vi "Handle MES commands.vi"(6 "Sequence Context In":refnum<k7>, 8 "error in (no error)":errorcluster, 9 "RequestData in":T2, 10 "Request":u32, 11 "Data Value Reference in":T1) -> (0 "error out":errorcluster, 1 "PLC MES Error":bool, 2 "RequestData out":T2, 3 "Data Value Reference out":T1)   [LabVIEW 2023]
uses:
  RequestData.ctl
  MessageInfo.ctl
  <vilib>/Noffz/UTP IO/UTP IO Library/methods/poly/plc/Write PLC Variable (Boolean).vi
  <vilib>/Noffz/UTP IO/UTP IO Library/methods/poly/plc/Read PLC Variable (String).vi
  <vilib>/addons/TestStand/_TSUtility.llb/TestStand - Get Property Value (String).vi
  <vilib>/addons/TestStand/_TSUtility.llb/TestStand - Set Property Value (String).vi
  <vilib>/addons/TestStand/_TSUtility.llb/TestStand - Set Property Value (Boolean).vi
  <vilib>/addons/TestStand/_TSUtility.llb/TestStand - Set Property Value (String Array).vi
  <vilib>/Noffz/UTP IO/UTP IO Library/UTP IO Pool Session.lvclass
  <vilib>/Noffz/UTP IO/UTP IO Library/methods/poly/plc/Write PLC Variable (String).vi
  <vilib>/Noffz/UTP IO/UTP IO Library/Typedefs/Session Handle.ctl
panel:
  out "Packaging Instructions":string[](array[string])
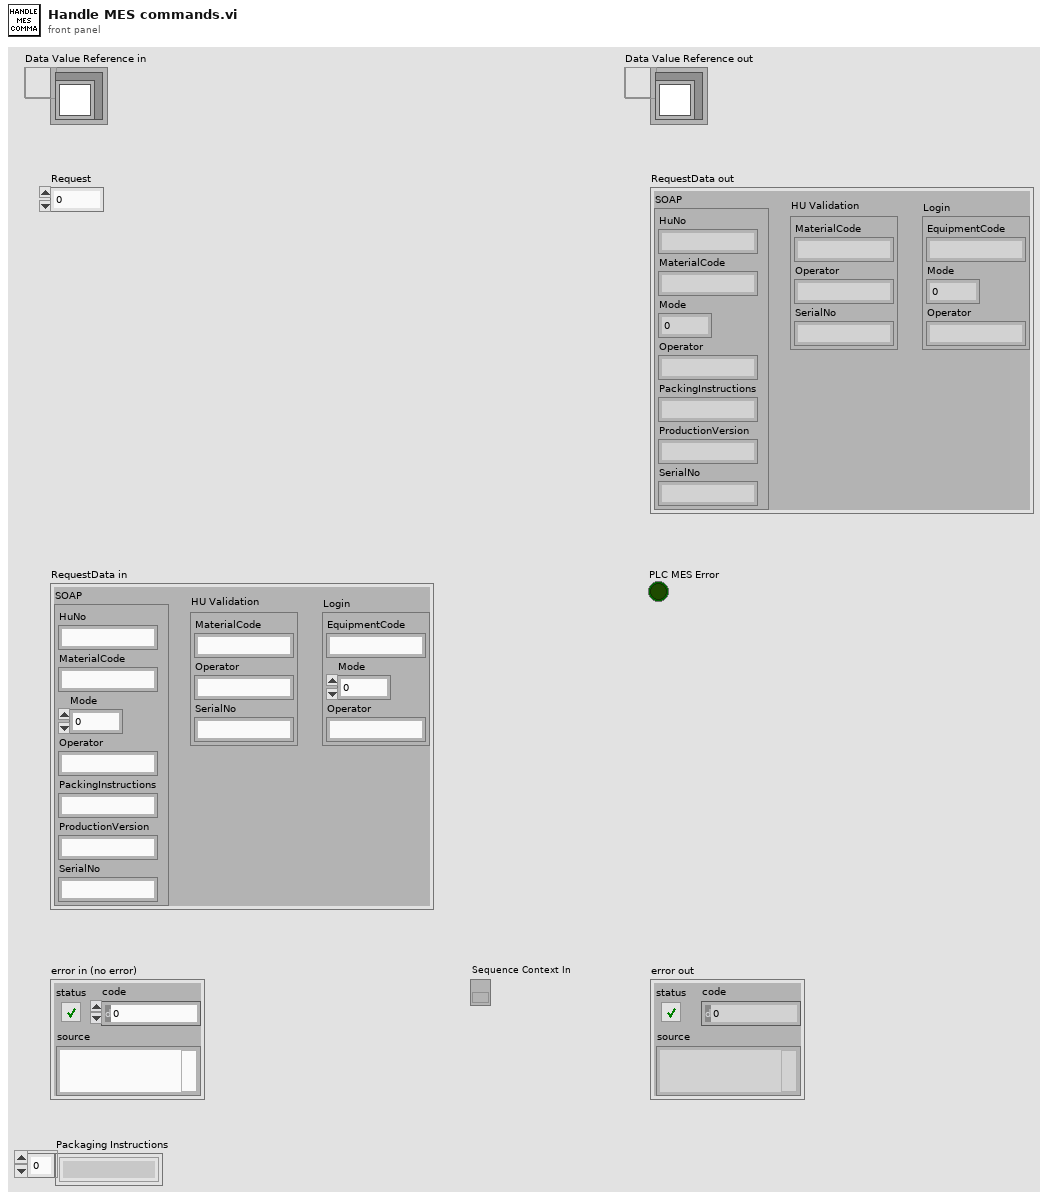
[diagram p1: front panel]
types:
  T1 = typedef "UTP IO Library.lvlib/UTP IO Pool Session.lvclass/Session Handle.ctl" = refnum<data-value>
  T2 = typedef "RequestData.ctl" = cluster{"SOAP":cluster{"HuNo":string, "MaterialCode":string, "Mode":i32, "Operator":string, "PackingInstructions":string, "ProductionVersion":string, "SerialNo":string}, "HU Validation":cluster{"MaterialCode":string, "Operator":string, "SerialNo":string}, "Login":cluster{"EquipmentCode":string, "Mode":i32, "Operator":string}}
  T3 = typedef "MessageInfo.ctl" = cluster{"Message Code":string, "Message Description":string}
  T4 = cluster{"EquipmentCode":string, "Mode":i32, "Operator":string}
  T5 = cluster{"MessageCode":string, "MessageDescription":string, "Result":string}
  T6 = cluster{"HuNo":string, "MaterialCode":string, "Mode":i32, "Operator":string, "PackingInstructions":string, "ProductionVersion":string, "SerialNo":string}
  T7 = cluster{"BoxCount":i32, "BoxNo":string, "MaxBoxCount":i32, "MaxSerialCount":i32, "MessageCode":string, "MessageDescription":string, "PackingInstruction1":string, "PackingInstruction2":string, "PackingInstruction3":string, "PackingInstruction4":string, "PackingInstruction5":string, "PalletNo":string, "Result":string, "SerialCount":i32}
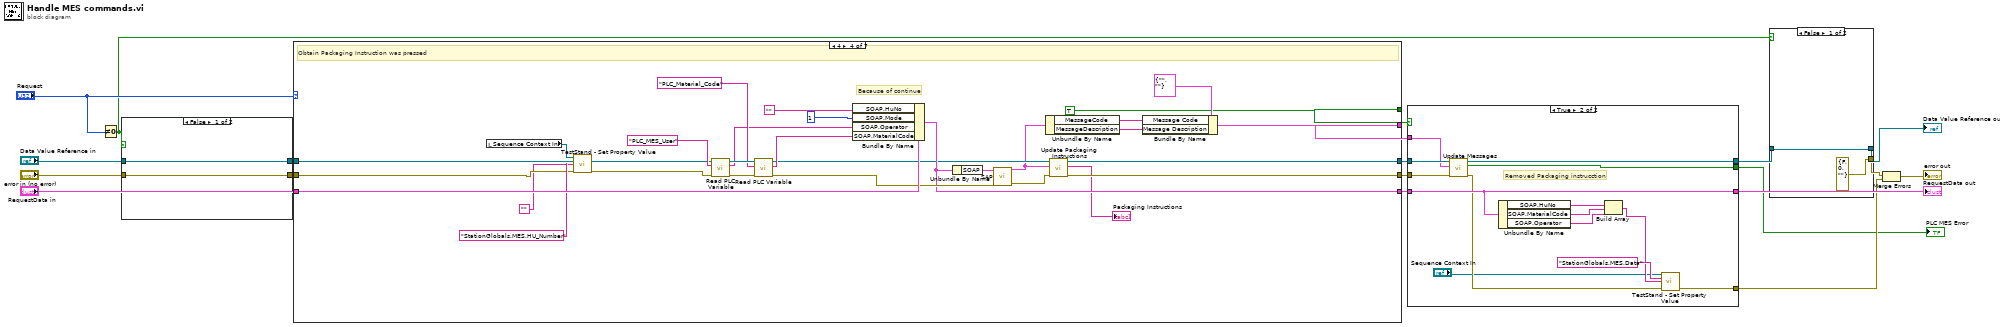
[diagram p0: block diagram]
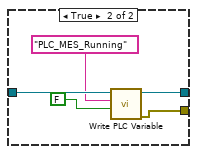
[diagram p2: hidden frame]
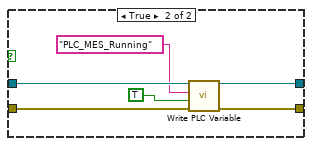
[diagram p3: hidden frame]
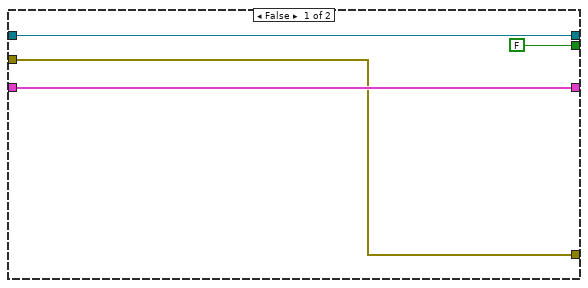
[diagram p4: hidden frame]
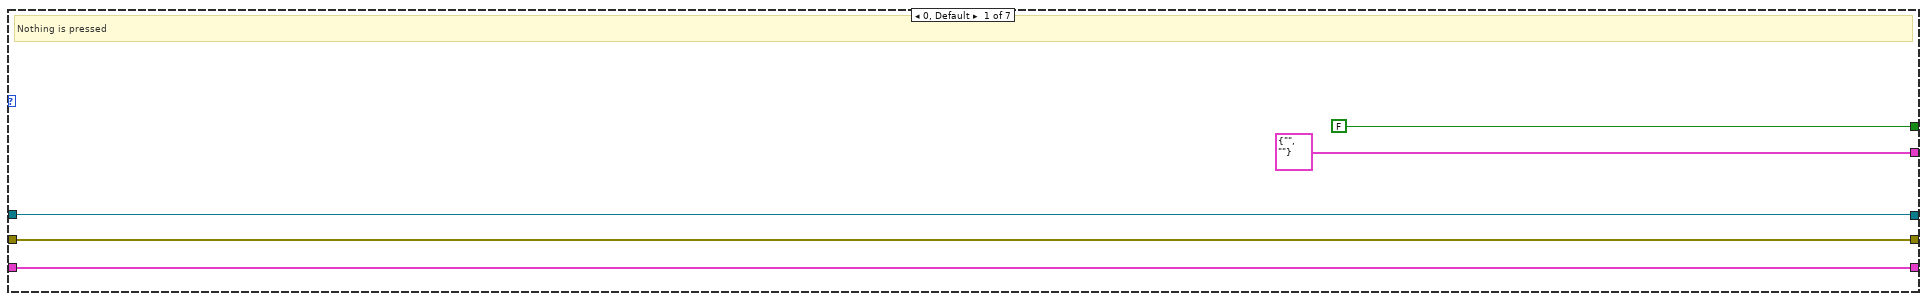
[diagram p5: hidden frame]
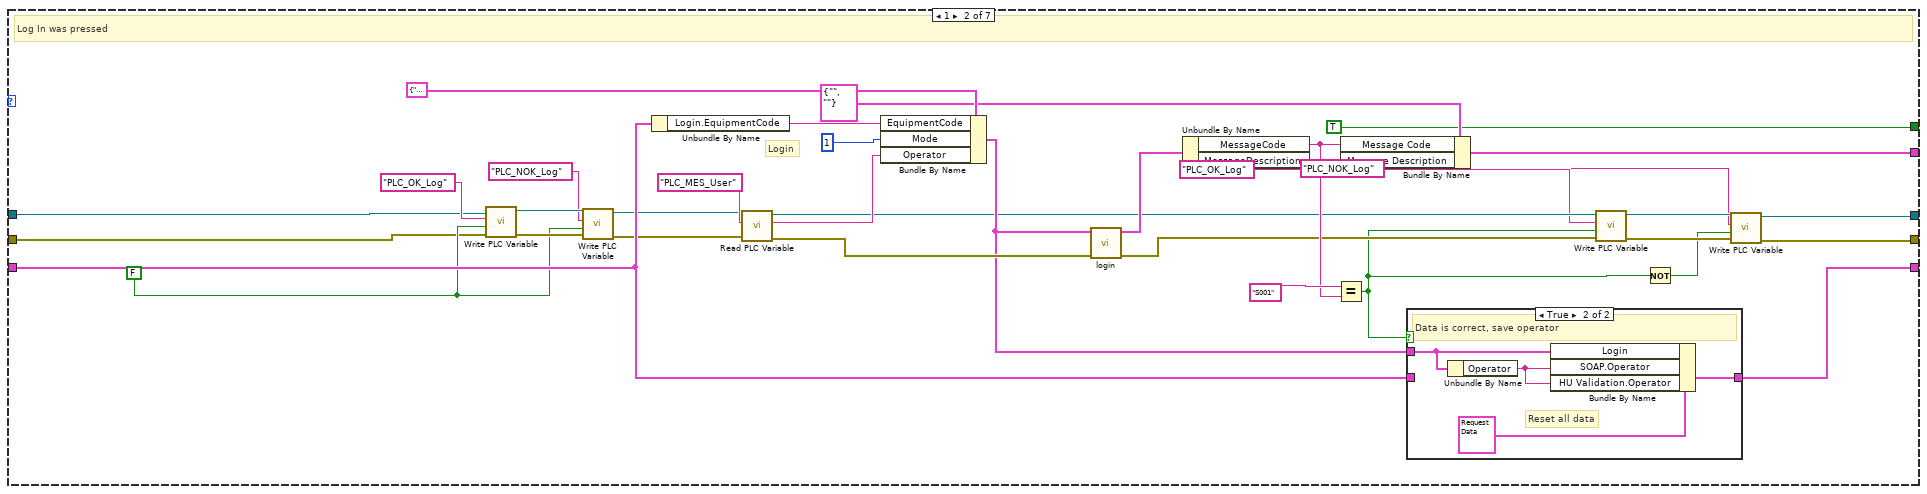
[diagram p6: hidden frame]
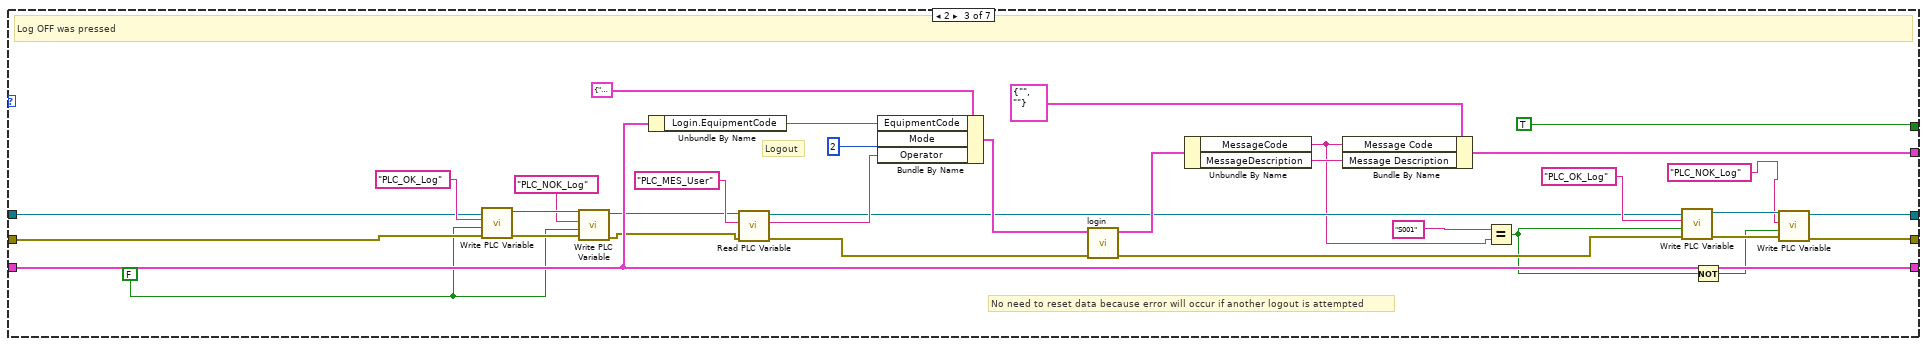
[diagram p8: hidden frame]
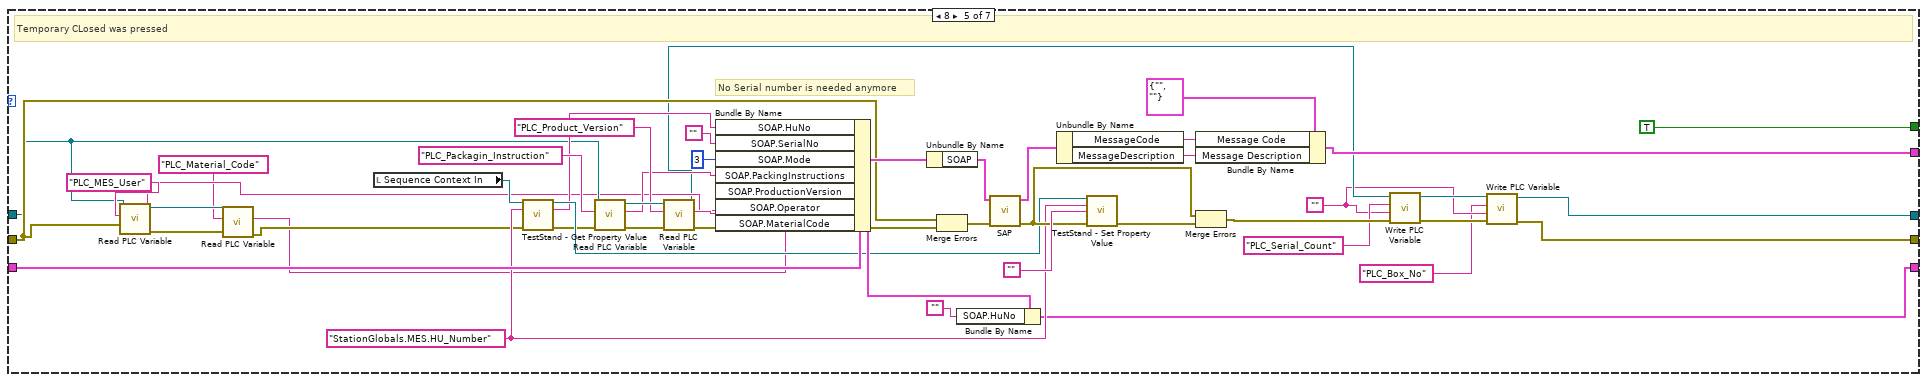
[diagram p9: hidden frame]
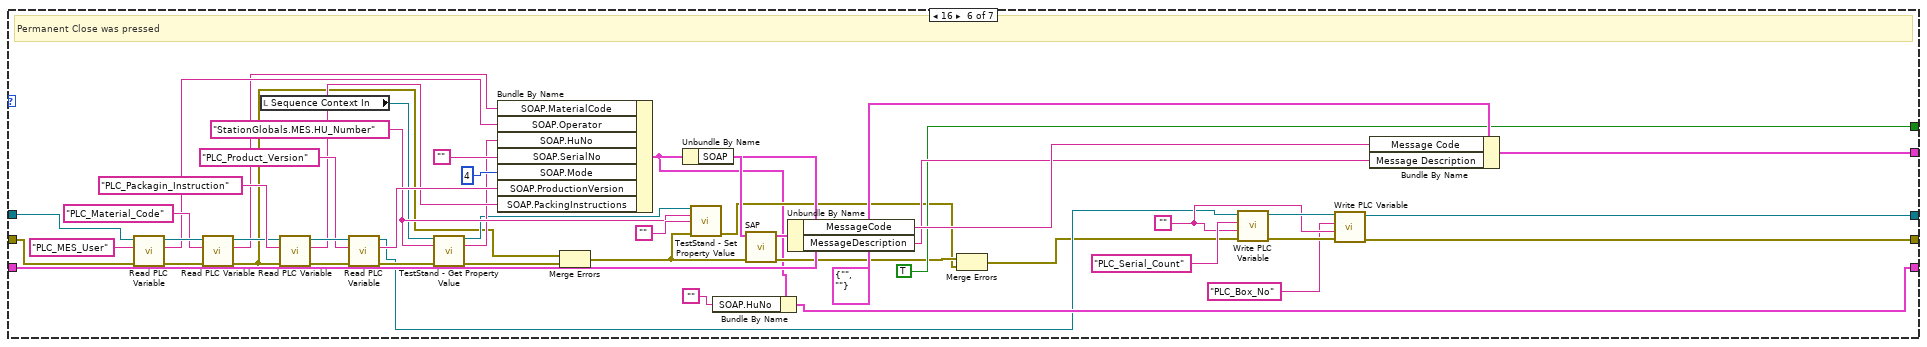
[diagram p10: hidden frame]
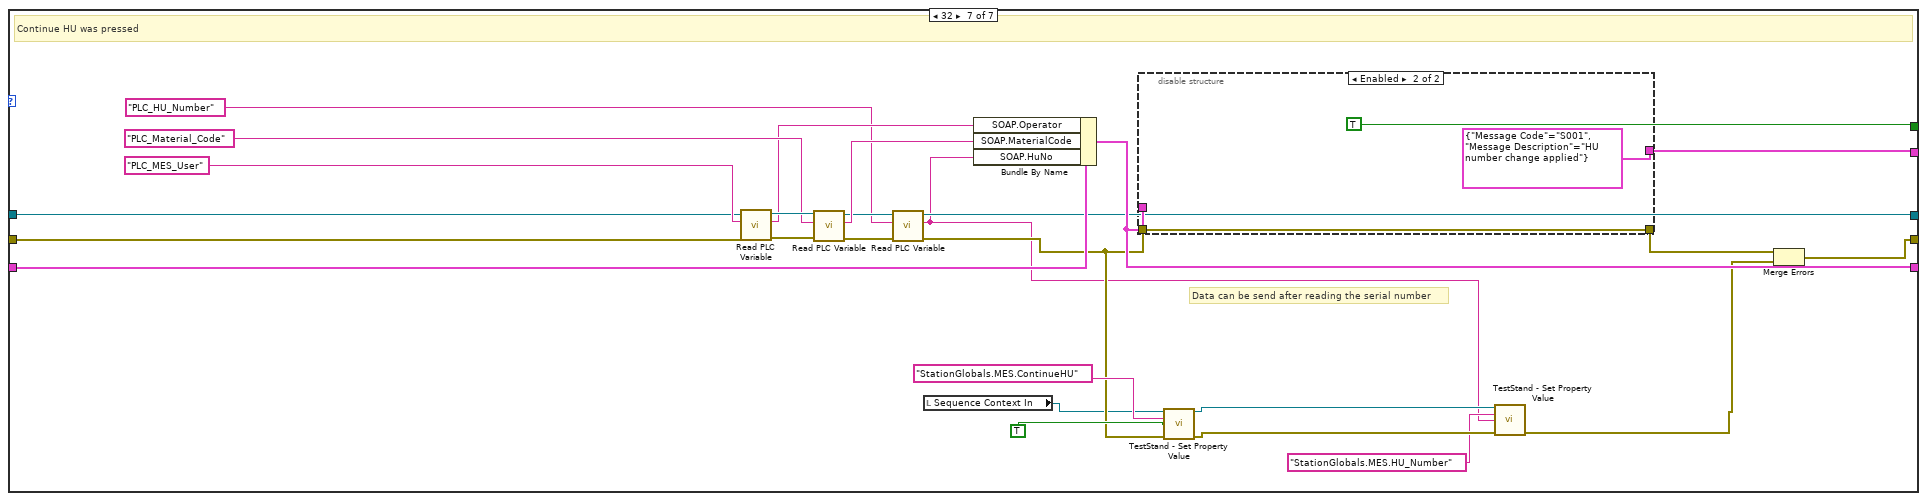
[diagram p11: hidden frame]
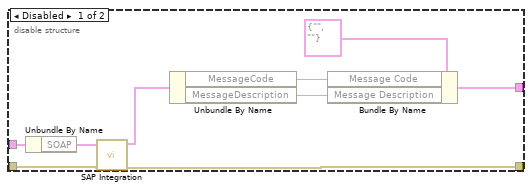
[diagram p12: hidden frame]
diagram:
  n1 = Not Equal To 0?(x="Request") -> (x != 0?=w5:bool)
  n2 = case shown="False" w5 {
    tunnel: "Data Value Reference in" -> [w21 w27]
    tunnel: [w21 w26] -> w11
    tunnel: "error in (no error)" -> [w20 w25]
    tunnel: [w20 w24] -> w9
    frame False {
    }
    frame True {
      n3 = call-poly <vilib>:"Write PLC Variable.vi"("error in (no error)"=w25, "value"=TRUE, "variable name"="PLC_MES_Running", "UTP IO Session in"=w27) -> ("error out"=w24:errorcluster, "UTP IO Session out"=w26:T1)  [unwired: 6 in]
    }
  }
  n4 = case shown="4" "Request" {
    tunnel: w9 -> [w28 w36 w75 w109 w152 w196 w250]
    tunnel: [w28 w45 w88 w120 w136 w184 w237] -> w17
    tunnel: w11 -> [w32 w35 w78 w131 w151 w198 w251]
    tunnel: [w32 w47 w89 w122 w140 w183 w245] -> w18
    tunnel: "RequestData in" -> [w29 w57 w99 w130 w182 w228 w249]
    tunnel: [w29 w61 w99 w126 w155 w203 w248] -> w14
    tunnel: [T3 {"Message Code"="", "Message Description"=""} w53 w95 w115 w174 w223 w243] -> w16
    tunnel: [FALSE TRUE TRUE TRUE TRUE TRUE TRUE] -> w15
    frame 0, Default {
      # "Nothing is pressed"
    }
    frame 1 {
      w38 = FALSE
      # "Login"
      # "Log In was pressed"
      n5 = call-poly <vilib>:"Write PLC Variable.vi"("error in (no error)"=w36, "value"=w38, "variable name"="PLC_OK_Log", "UTP IO Session in"=w35) -> ("error out"=w39:errorcluster, "UTP IO Session out"=w40:T1)  [unwired: 6 in]
      n6 = call-poly <vilib>:"Write PLC Variable.vi"("error in (no error)"=w39, "value"=w38, "variable name"="PLC_NOK_Log", "UTP IO Session in"=w40) -> ("error out"=w33:errorcluster, "UTP IO Session out"=w34:T1)  [unwired: 6 in]
      n7 = Unbundle By Name(w57) -> ("Login.EquipmentCode"=w62:string)
      n8 = call-poly <vilib>:"Read PLC Variable.vi"("error in (no error)"=w33, "variable name"="PLC_MES_User", "UTP IO Session in"=w34) -> ("error out"=w66:errorcluster, "value"=w64:string, "UTP IO Session out"=w51:T1)  [unwired: 6 in]
      n9 = Bundle By Name(cluster=T4 {"EquipmentCode"="", "Mode"=0, "Operator"=""} ("Login Input"), "EquipmentCode"=w62, "Mode"=1, "Operator"=w64) -> (w60:T4)
      n10 = call "login.vi"("error in (no error)"=w66, "in"=w60) -> ("error out"=w50:errorcluster, "out"=w59:T5)  [unwired: 8 in]
      n11 = Unbundle By Name(w59) -> ("MessageCode"=w55:string, "MessageDescription"=w54:string)
      n12 = Equal?(x="S001", y=w55) -> (x = y?=w43:bool)
      n13 = Bundle By Name(cluster=T3 {"Message Code"="", "Message Description"=""}, "Message Code"=w55, "Message Description"=w54) -> (w53:T3)
      n14 = case shown="True" w43 {
        tunnel: [w68 w72] -> w61
        tunnel: w60 -> [_ w70]
        tunnel: w57 -> [w68 _]
        frame False {
          # "Remember old data because there was an error"
        }
        frame True {
          # "Reset all data"
          # "Data is correct, save operator"
          n15 = Unbundle By Name(w70) -> ("Operator"=w69:string)
          n16 = Bundle By Name(cluster=T2 {"SOAP"={"HuNo"="", "MaterialCode"="", "Mode"=0, "Operator"="", "PackingInstructions"="", "ProductionVersion"="", "SerialNo"=""}, "HU Validation"={"MaterialCode"="", "Operator"="", "SerialNo"=""}, "Login"={"EquipmentCode"="", "Mode"=0, "Operator"=""}} ("RequestData in 2"), "Login"=w70, "SOAP.Operator"=w69, "HU Validation.Operator"=w69) -> (w72:T2)
        }
      }
      n17 = call-poly <vilib>:"Write PLC Variable.vi"("error in (no error)"=w50, "value"=w43, "variable name"="PLC_OK_Log", "UTP IO Session in"=w51) -> ("error out"=w46:errorcluster, "UTP IO Session out"=w48:T1)  [unwired: 6 in]
      n18 = Not(x=w43) -> (.not. x?=w42:bool)
      n19 = call-poly <vilib>:"Write PLC Variable.vi"("error in (no error)"=w46, "value"=w42, "variable name"="PLC_NOK_Log", "UTP IO Session in"=w48) -> ("error out"=w45:errorcluster, "UTP IO Session out"=w47:T1)  [unwired: 6 in]
    }
    frame 2 {
      w74 = FALSE
      # "No need to reset data because error will occur if another logout is attempted"
      # "Logout"
      # "Log OFF was pressed"
      n20 = call-poly <vilib>:"Write PLC Variable.vi"("error in (no error)"=w75, "value"=w74, "variable name"="PLC_OK_Log", "UTP IO Session in"=w78) -> ("error out"=w79:errorcluster, "UTP IO Session out"=w80:T1)  [unwired: 6 in]
      n21 = call-poly <vilib>:"Write PLC Variable.vi"("error in (no error)"=w79, "value"=w74, "variable name"="PLC_NOK_Log", "UTP IO Session in"=w80) -> ("error out"=w76:errorcluster, "UTP IO Session out"=w77:T1)  [unwired: 6 in]
      n22 = Unbundle By Name(w99) -> ("Login.EquipmentCode"=w101:string)
      n23 = call-poly <vilib>:"Read PLC Variable.vi"("error in (no error)"=w76, "variable name"="PLC_MES_User", "UTP IO Session in"=w77) -> ("error out"=w105:errorcluster, "value"=w103:string, "UTP IO Session out"=w86:T1)  [unwired: 6 in]
      n24 = Bundle By Name(cluster=T4 {"EquipmentCode"="", "Mode"=0, "Operator"=""} ("Login Input"), "EquipmentCode"=w101, "Mode"=2, "Operator"=w103) -> (w100:T4)
      n25 = call "login.vi"("error in (no error)"=w105, "in"=w100) -> ("error out"=w85:errorcluster, "out"=w96:T5)  [unwired: 8 in]
      n26 = Unbundle By Name(w96) -> ("MessageCode"=w83:string, "MessageDescription"=w97:string)
      n27 = Bundle By Name(cluster=T3 {"Message Code"="", "Message Description"=""}, "Message Code"=w83, "Message Description"=w97) -> (w95:T3)
      n28 = Equal?(x="S001", y=w83) -> (x = y?=w82:bool)
      n29 = call-poly <vilib>:"Write PLC Variable.vi"("error in (no error)"=w85, "value"=w82, "variable name"="PLC_OK_Log", "UTP IO Session in"=w86) -> ("error out"=w91:errorcluster, "UTP IO Session out"=w92:T1)  [unwired: 6 in]
      n30 = Not(x=w82) -> (.not. x?=w90:bool)
      n31 = call-poly <vilib>:"Write PLC Variable.vi"("error in (no error)"=w91, "value"=w90, "variable name"="PLC_NOK_Log", "UTP IO Session in"=w92) -> ("error out"=w88:errorcluster, "UTP IO Session out"=w89:T1)  [unwired: 6 in]
    }
    frame 4 {
      # "Because of continue"
      # "Obtain Packaging Instruction was pressed"
      n32 = local read "Sequence Context In"() -> (w111:refnum<k7>)
      n33 = call-poly <vilib>:"TestStand - Set Property Value.vi"("Sequence Context In"=w111, "Lookup String"="StationGlobals.MES.HU_Number", "New Value"="", "error in (no error)"=w109) -> ("error out"=w108:errorcluster)  [unwired: 10 in, 1 out]
      n34 = call-poly <vilib>:"Read PLC Variable.vi"("error in (no error)"=w108, "variable name"="PLC_MES_User", "UTP IO Session in"=w131) -> ("error out"=w133:errorcluster, "value"=w128:string, "UTP IO Session out"=w134:T1)  [unwired: 6 in]
      n35 = call-poly <vilib>:"Read PLC Variable.vi"("error in (no error)"=w133, "variable name"="PLC_Material_Code", "UTP IO Session in"=w134) -> ("error out"=w129:errorcluster, "value"=w127:string, "UTP IO Session out"=w123:T1)  [unwired: 6 in]
      n36 = Bundle By Name(cluster=w130, "SOAP.HuNo"="", "SOAP.Mode"=1, "SOAP.Operator"=w128, "SOAP.MaterialCode"=w127) -> (w126:T2)
      n37 = Unbundle By Name(w126) -> ("SOAP"=w125:T6)
      n38 = call "SAP.vi"("error in (no error)"=w129, "input"=w125) -> ("error out"=w121:errorcluster, "output"=w118:T7)  [unwired: 8 in]
      n39 = Unbundle By Name(w118) -> ("MessageCode"=w117:string, "MessageDescription"=w116:string)
      n40 = call "Update Packaging Instructions.vi"("error in (no error)"=w121, "Output Parameters"=w118, "Data Value Reference in"=w123) -> ("error out"=w120:errorcluster, "Packaging Instructions"=→"Packaging Instructions":string[], "Data Value Reference out"=w122:T1)  [unwired: 6 in]
      n41 = Bundle By Name(cluster=T3 {"Message Code"="", "Message Description"=""}, "Message Code"=w117, "Message Description"=w116) -> (w115:T3)
    }
    frame 8 {
      w138 = ""
      w159 = "StationGlobals.MES.HU_Number" ("Lookup String")
      # "No Serial number is needed anymore"
      # "Temporary CLosed was pressed"
      n42 = call-poly <vilib>:"Read PLC Variable.vi"("error in (no error)"=w152, "variable name"="PLC_MES_User", "UTP IO Session in"=w151) -> ("error out"=w149:errorcluster, "value"=w150:string, "UTP IO Session out"=w147:T1)  [unwired: 6 in]
      n43 = call-poly <vilib>:"Read PLC Variable.vi"("error in (no error)"=w149, "variable name"="PLC_Material_Code", "UTP IO Session in"=w147) -> ("error out"=w148:errorcluster, "value"=w145:string)  [unwired: 6 in, 1 out]
      n44 = local read "Sequence Context In"() -> (w161:refnum<k7>)
      n45 = call-poly <vilib>:"TestStand - Get Property Value.vi"("Sequence Context In"=w161, "Lookup String"=w159, "error in (no error)"=w148) -> ("Sequence Context Out"=w160:refnum<k7>, "Value"=w156:string, "error out"=w158:errorcluster)  [unwired: 10 in]
      n46 = call-poly <vilib>:"Read PLC Variable.vi"("error in (no error)"=w158, "variable name"="PLC_Packagin_Instruction", "UTP IO Session in"=w151) -> ("error out"=w168:errorcluster, "value"=w163:string, "UTP IO Session out"=w169:T1)  [unwired: 6 in]
      n47 = call-poly <vilib>:"Read PLC Variable.vi"("error in (no error)"=w168, "variable name"="PLC_Product_Version", "UTP IO Session in"=w169) -> ("error out"=w164:errorcluster, "value"=w162:string, "UTP IO Session out"=w143:T1)  [unwired: 6 in]
      n48 = Bundle By Name(cluster=w182, "SOAP.HuNo"=w156, "SOAP.SerialNo"="", "SOAP.Mode"=3, "SOAP.PackingInstructions"=w163, "SOAP.ProductionVersion"=w162, "SOAP.Operator"=w150, "SOAP.MaterialCode"=w145) -> (w181:T2)
      n49 = Unbundle By Name(w181) -> ("SOAP"=w179:T6)
      n50 = Merge Errors(w152, w164) -> (w165:errorcluster)
      n51 = Bundle By Name(cluster=w181, "SOAP.HuNo"="") -> (w155:T2)
      n52 = call "SAP.vi"("error in (no error)"=w165, "input"=w179) -> ("error out"=w171:errorcluster, "output"=w175:T7)  [unwired: 8 in]
      n53 = Unbundle By Name(w175) -> ("MessageCode"=w177:string, "MessageDescription"=w176:string)
      n54 = call-poly <vilib>:"TestStand - Set Property Value.vi"("Sequence Context In"=w160, "Lookup String"=w159, "New Value"="", "error in (no error)"=w171) -> ("error out"=w170:errorcluster)  [unwired: 10 in, 1 out]
      n55 = Bundle By Name(cluster=T3 {"Message Code"="", "Message Description"=""}, "Message Code"=w177, "Message Description"=w176) -> (w174:T3)
      n56 = Merge Errors(w171, w170) -> (w144:errorcluster)
      n57 = call-poly <vilib>:"Write PLC Variable.vi"("error in (no error)"=w144, "value"=w138, "variable name"="PLC_Serial_Count", "UTP IO Session in"=w143) -> ("error out"=w142:errorcluster, "UTP IO Session out"=w141:T1)  [unwired: 6 in]
      n58 = call-poly <vilib>:"Write PLC Variable.vi"("error in (no error)"=w142, "value"=w138, "variable name"="PLC_Box_No", "UTP IO Session in"=w141) -> ("error out"=w136:errorcluster, "UTP IO Session out"=w140:T1)  [unwired: 6 in]
    }
    frame 16 {
      w188 = ""
      w208 = "StationGlobals.MES.HU_Number" ("Lookup String")
      # "Permanent Close was pressed"
      n59 = call-poly <vilib>:"Read PLC Variable.vi"("error in (no error)"=w196, "variable name"="PLC_MES_User", "UTP IO Session in"=w198) -> ("error out"=w200:errorcluster, "value"=w193:string, "UTP IO Session out"=w199:T1)  [unwired: 6 in]
      n60 = call-poly <vilib>:"Read PLC Variable.vi"("error in (no error)"=w200, "variable name"="PLC_Material_Code", "UTP IO Session in"=w199) -> ("error out"=w195:errorcluster, "value"=w192:string, "UTP IO Session out"=w197:T1)  [unwired: 6 in]
      n61 = local read "Sequence Context In"() -> (w207:refnum<k7>)
      n62 = call-poly <vilib>:"Read PLC Variable.vi"("error in (no error)"=w195, "variable name"="PLC_Packagin_Instruction", "UTP IO Session in"=w197) -> ("error out"=w217:errorcluster, "value"=w212:string, "UTP IO Session out"=w218:T1)  [unwired: 6 in]
      n63 = call-poly <vilib>:"Read PLC Variable.vi"("error in (no error)"=w217, "variable name"="PLC_Product_Version", "UTP IO Session in"=w218) -> ("error out"=w210:errorcluster, "value"=w213:string, "UTP IO Session out"=w186:T1)  [unwired: 6 in]
      n64 = call-poly <vilib>:"TestStand - Get Property Value.vi"("Sequence Context In"=w207, "Lookup String"=w208, "error in (no error)"=w210) -> ("Sequence Context Out"=w205:refnum<k7>, "Value"=w206:string, "error out"=w209:errorcluster)  [unwired: 10 in]
      n65 = Bundle By Name(cluster=w228, "SOAP.MaterialCode"=w192, "SOAP.Operator"=w193, "SOAP.HuNo"=w206, "SOAP.SerialNo"="", "SOAP.Mode"=4, "SOAP.ProductionVersion"=w213, "SOAP.PackingInstructions"=w212) -> (w204:T2)
      n66 = Merge Errors(w195, w209) -> (w214:errorcluster)
      n67 = Unbundle By Name(w204) -> ("SOAP"=w229:T6)
      n68 = call-poly <vilib>:"TestStand - Set Property Value.vi"("Sequence Context In"=w205, "Lookup String"=w208, "New Value"="", "error in (no error)"=w214) -> ("error out"=w220:errorcluster)  [unwired: 10 in, 1 out]
      n69 = Bundle By Name(cluster=w204, "SOAP.HuNo"="") -> (w203:T2)
      n70 = call "SAP.vi"("error in (no error)"=w214, "input"=w229) -> ("error out"=w221:errorcluster, "output"=w224:T7)  [unwired: 8 in]
      n71 = Unbundle By Name(w224) -> ("MessageCode"=w226:string, "MessageDescription"=w225:string)
      n72 = Merge Errors(w221, w220) -> (w185:errorcluster)
      n73 = call-poly <vilib>:"Write PLC Variable.vi"("error in (no error)"=w185, "value"=w188, "variable name"="PLC_Serial_Count", "UTP IO Session in"=w186) -> ("error out"=w191:errorcluster, "UTP IO Session out"=w190:T1)  [unwired: 6 in]
      n74 = call-poly <vilib>:"Write PLC Variable.vi"("error in (no error)"=w191, "value"=w188, "variable name"="PLC_Box_No", "UTP IO Session in"=w190) -> ("error out"=w184:errorcluster, "UTP IO Session out"=w183:T1)  [unwired: 6 in]
      n75 = Bundle By Name(cluster=T3 {"Message Code"="", "Message Description"=""}, "Message Code"=w226, "Message Description"=w225) -> (w223:T3)
    }
    frame 32 {
      # "Data can be send after reading the serial number"
      # "Continue HU was pressed"
      n76 = call-poly <vilib>:"Read PLC Variable.vi"("error in (no error)"=w250, "variable name"="PLC_MES_User", "UTP IO Session in"=w251) -> ("error out"=w255:errorcluster, "value"=w253:string, "UTP IO Session out"=w256:T1)  [unwired: 6 in]
      n77 = call-poly <vilib>:"Read PLC Variable.vi"("error in (no error)"=w255, "variable name"="PLC_Material_Code", "UTP IO Session in"=w256) -> ("error out"=w247:errorcluster, "value"=w252:string, "UTP IO Session out"=w246:T1)  [unwired: 6 in]
      n78 = call-poly <vilib>:"Read PLC Variable.vi"("error in (no error)"=w247, "variable name"="PLC_HU_Number", "UTP IO Session in"=w246) -> ("error out"=w239:errorcluster, "value"=w231:string, "UTP IO Session out"=w245:T1)  [unwired: 6 in]
      n79 = local read "Sequence Context In"() -> (w236:refnum<k7>)
      n80 = Bundle By Name(cluster=w249, "SOAP.Operator"=w253, "SOAP.MaterialCode"=w252, "SOAP.HuNo"=w231) -> (w248:T2)
      n81 = disable-structure shown="Enabled" {
        disable-tunnel: [w265 w268] -> w238
        disable-tunnel: w248 -> [w264 _]
        disable-tunnel: w239 -> [w259 w268]
        disable-tunnel: [w258 T3 {"Message Code"="S001", "Message Description"="HU number change applied"}] -> w243
        frame Disabled {
          n82 = Unbundle By Name(w264) -> ("SOAP"=w266:T6)
          n83 = call "SAP Integration.vi"("error in"=w259, "Input Parameters"=w266) -> ("error out"=w265:errorcluster, "Output Parameters"=w260:T7)  [unwired: 8 in]
          n84 = Unbundle By Name(w260) -> ("MessageCode"=w262:string, "MessageDescription"=w261:string)
          n85 = Bundle By Name(cluster=T3 {"Message Code"="", "Message Description"=""}, "Message Code"=w262, "Message Description"=w261) -> (w258:T3)
        }
        frame Enabled {
        }
      }
      n86 = call-poly <vilib>:"TestStand - Set Property Value.vi"("Sequence Context In"=w236, "Lookup String"="StationGlobals.MES.ContinueHU", "New Value"=TRUE, "error in (no error)"=w239) -> ("Sequence Context Out"=w235:refnum<k7>, "error out"=w234:errorcluster)  [unwired: 10 in]
      n87 = call-poly <vilib>:"TestStand - Set Property Value.vi"("Sequence Context In"=w235, "Lookup String"="StationGlobals.MES.HU_Number", "New Value"=w231, "error in (no error)"=w234) -> ("error out"=w233:errorcluster)  [unwired: 10 in, 1 out]
      n88 = Merge Errors(w238, w233) -> (w237:errorcluster)
    }
  }
  n89 = case shown="True" w15 {
    tunnel: [w272 w286] -> w8
    tunnel: w18 -> [w272 w285]
    tunnel: w17 -> [w270 w284]
    tunnel: w16 -> [_ w283]
    tunnel: w14 -> [w271 w278]
    tunnel: [w271 w278] -> w13
    tunnel: [w270 w274] -> w2
    tunnel: [FALSE ("PLC MES Error") w273] -> w1
    frame False {
    }
    frame True {
      # "Removed Packaging instrucction"
      n90 = call "Update Messages.vi"("error in (no error)"=w284, "Message Info"=w283, "Data Value Reference in"=w285) -> ("error out"=w276:errorcluster, "PLC MES Error"=w273:bool, "Data Value Reference out"=w286:T1)  [unwired: 6 in]
      n91 = Unbundle By Name(w278) -> ("SOAP.HuNo"=w282:string, "SOAP.MaterialCode"=w281:string, "SOAP.Operator"=w280:string)
      n92 = Build Array(w282, w281, w280) -> (w277:string[])
      n93 = call-poly <vilib>:"TestStand - Set Property Value.vi"("Sequence Context In"="Sequence Context In", "Lookup String"="StationGlobals.MES.Data", "New Value"=w277, "error in (no error)"=w276) -> ("error out"=w274:errorcluster)  [unwired: 10 in, 1 out]
    }
  }
  "RequestData out" <- w13
  "PLC MES Error" <- w1
  n94 = case shown="False" w5 {
    tunnel: w8 -> [w288 w292]
    tunnel: [w288 w291] -> w7
    tunnel: [errorcluster {"status"=FALSE, "code"=0, "source"=""} ("error out") w289] -> w4
    frame False {
    }
    frame True {
      n95 = call-poly <vilib>:"Write PLC Variable.vi"("value"=FALSE, "variable name"="PLC_MES_Running", "UTP IO Session in"=w292) -> ("error out"=w289:errorcluster, "UTP IO Session out"=w291:T1)  [unwired: 7 in]
    }
  }
  "Data Value Reference out" <- w7
  n96 = Merge Errors(w4, w2) -> (→"error out":errorcluster)
